vi "asdfghjkl.vi"() -> ()   [LabVIEW 2017]
panel:
  in  "Boolean array":bool[](array[boolean])
  out "Slide":i8(slide) scale=0.0..15.0 scale format="%x"
  in  "stop 2":bool
  out "Boolean 13":bool
  out "Boolean 12":bool
  out "Boolean 11":bool
  out "Boolean 10":bool
  out "Boolean 9":bool
  out "Boolean 8":bool
  out "Boolean 7":bool
  in  "stop":bool
  out "Boolean 6":bool
  out "Boolean 5":bool
  in  "Boolean 4":bool
  in  "Boolean 3":bool
  in  "Boolean 2":bool
  in  "Boolean":bool
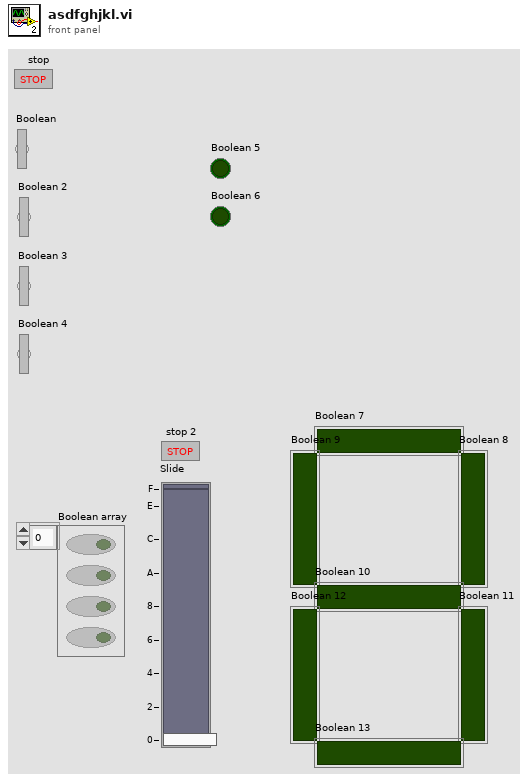
[diagram p1: front panel]
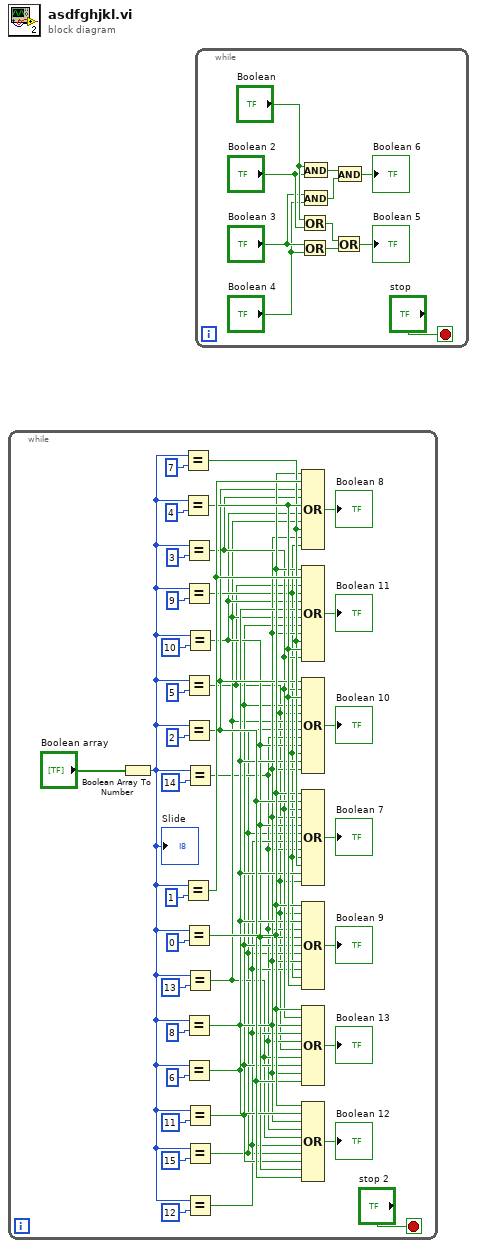
[diagram p0: block diagram]
diagram:
  n1 = while {
    stop <- "stop 2" stop-if-true
    n2 = Boolean Array To Number(Boolean array="Boolean array") -> (number=w8:u32)
    "Slide" <- w8
    n3 = Equal?(x=w8, y=i8 7) -> (x = y?=w22:bool)
    n4 = Equal?(x=w8, y=i8 4) -> (x = y?=w23:bool)
    n5 = Equal?(x=w8, y=i8 1) -> (x = y?=w24:bool)
    n6 = Equal?(x=w8, y=i8 3) -> (x = y?=w19:bool)
    n7 = Equal?(x=w8, y=i8 9) -> (x = y?=w16:bool)
    n8 = Equal?(x=w8, y=i8 5) -> (x = y?=w1:bool)
    n9 = Equal?(x=w8, y=i8 2) -> (x = y?=w20:bool)
    n10 = Equal?(x=w8, y=i8 0) -> (x = y?=w21:bool)
    n11 = Equal?(x=w8, y=i8 8) -> (x = y?=w17:bool)
    n12 = Equal?(x=w8, y=i8 6) -> (x = y?=w18:bool)
    n13 = Equal?(x=w8, y=i8 10) -> (x = y?=w7:bool)
    n14 = Equal?(x=w8, y=i8 14) -> (x = y?=w3:bool)
    n15 = Equal?(x=w8, y=i8 13) -> (x = y?=w4:bool)
    n16 = Equal?(x=w8, y=i8 11) -> (x = y?=w6:bool)
    n17 = Equal?(x=w8, y=i8 15) -> (x = y?=w2:bool)
    n18 = Equal?(x=w8, y=i8 12) -> (x = y?=w5:bool)
    n19 = Compound Arithmetic op=OR(w21, w24, w20, w19, w23, w7, w4, w22, w17, w16) -> (→"Boolean 8":bool)
    n20 = Compound Arithmetic op=OR(w21, w24, w1, w16, w7, w18, w4, w6, w17, w22, w23, w19) -> (→"Boolean 11":bool)
    n21 = Compound Arithmetic op=OR(w20, w19, w23, w6, w1, w4, w2, w3, w7, w16, w18, w17) -> (→"Boolean 10":bool)
    n22 = Compound Arithmetic op=OR(w21, w20, w19, w17, w7, w2, w5, w3, w16, w22, w18, w1) -> (→"Boolean 7":bool)
    n23 = Compound Arithmetic op=OR(w21, w1, w18, w3, w7, w6, w2, w17, w5, w16, w23) -> (→"Boolean 9":bool)
    n24 = Compound Arithmetic op=OR(w21, w19, w18, w5, w3, w1, w4, w6, w17, w20) -> (→"Boolean 13":bool)
    n25 = Compound Arithmetic op=OR(w21, w18, w17, w3, w4, w5, w2, w6, w7, w20) -> (→"Boolean 12":bool)
  }
  n26 = while {
    stop <- "stop" stop-if-true
    n27 = Or(x="Boolean", y="Boolean 2") -> (x .or. y?=w46:bool)
    n28 = Or(x="Boolean 3", y="Boolean 4") -> (x .or. y?=w45:bool)
    n29 = And(x="Boolean", y="Boolean 2") -> (x .and. y?=w52:bool)
    n30 = And(x="Boolean 3", y="Boolean 4") -> (x .and. y?=w53:bool)
    n31 = Or(x=w46, y=w45) -> (x .or. y?=→"Boolean 5":bool)
    n32 = And(x=w52, y=w53) -> (x .and. y?=→"Boolean 6":bool)
  }
